vi "test.vi"() -> ()   [LabVIEW 2023, in "Serial_communication.lvlib"]
uses:
  Serial_communication.lvlib
panel:
  out "Read value 2":string
  out "LED ON":bool
  in  "?":bool
  out "Read value":string
  in  "stop":bool
  in  "Command":string
  in  "?":bool
  out "error out":errorcluster
  in  "Visa resourse":refnum<visa-resource-name>
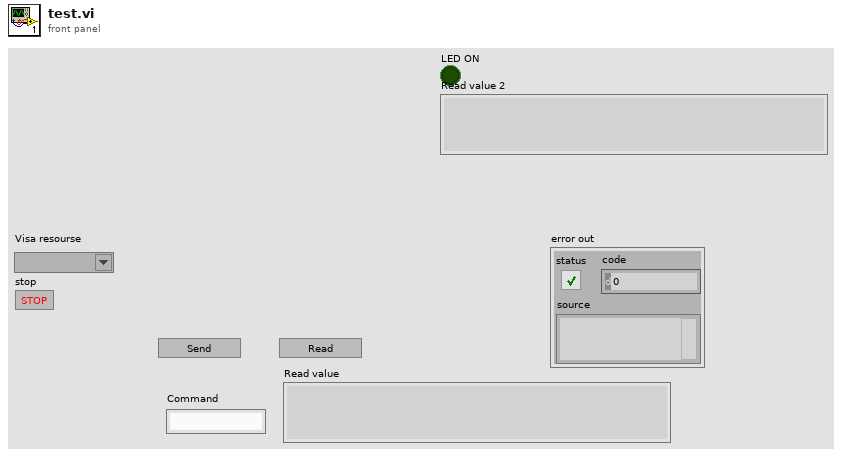
[diagram p1: front panel]
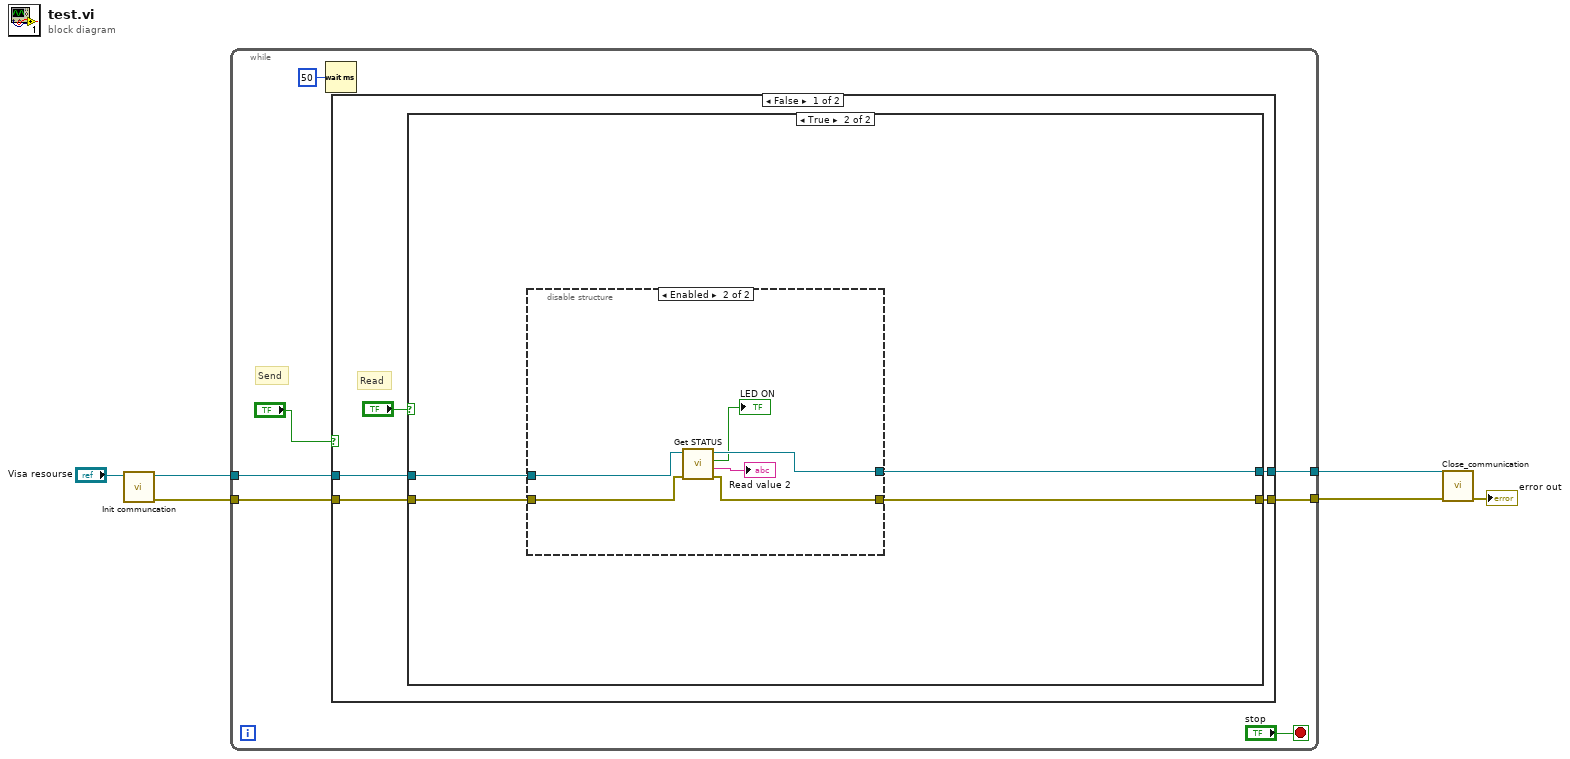
[diagram p0: block diagram]
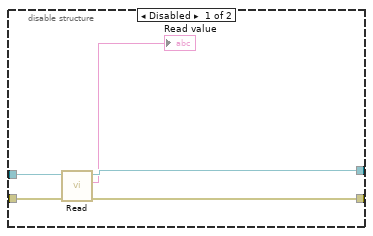
[diagram p3: hidden frame]
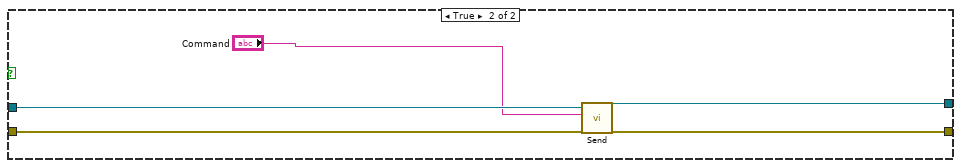
[diagram p4: hidden frame]
diagram:
  n1 = call "Init communcation.vi"("COM port"="Visa resourse") -> ("error out"=w3:errorcluster, "VISA Refnum out"=w4:refnum<visa-resource-name>)  [unwired: 9 in]
  n2 = while {
    tunnel: w4 -> [w12]
    tunnel: w3 -> [w11]
    tunnel: [w8] -> w2
    tunnel: [w7] -> w1
    stop <- "stop" stop-if-true
    # "Send"
    n3 = Wait (ms)(milliseconds to wait=u32 50) -> ()  [unwired: 1 out]
    n4 = case shown="False" "?" {
      tunnel: w12 -> [w18 w40]
      tunnel: w11 -> [w17 w39]
      tunnel: [w16 w38] -> w8
      tunnel: [w15 w37] -> w7
      frame False {
        # "Read"
        n5 = case shown="True" "?" {
          tunnel: w18 -> [w19 w24]
          tunnel: w17 -> [w20 w23]
          tunnel: [w19 w22] -> w16
          tunnel: [w20 w21] -> w15
          frame False {
          }
          frame True {
            n6 = disable-structure shown="Enabled" {
              disable-tunnel: w24 -> [w29 w35]
              disable-tunnel: w23 -> [w28 w34]
              disable-tunnel: [w27 w33] -> w22
              disable-tunnel: [w26 w32] -> w21
              frame Disabled {
                n7 = call "Read.vi"("error in (no error)"=w28, "VISA Refnum in"=w29) -> ("error out"=w26:errorcluster, "Read value"=→"Read value":string, "VISA Refnum out"=w27:refnum<visa-resource-name>)  [unwired: 7 in]
              }
              frame Enabled {
                n8 = call "Get STATUS.vi"("error in (no error)"=w34, "VISA Refnum in"=w35) -> ("error out"=w32:errorcluster, "Read value"=→"Read value 2":string, "LED ON"=→"LED ON":bool, "VISA Refnum out"=w33:refnum<visa-resource-name>)  [unwired: 6 in]
              }
            }
          }
        }
      }
      frame True {
        n9 = call "Send.vi"("error in (no error)"=w39, "Command"="Command", "VISA Refnum in"=w40) -> ("error out"=w37:errorcluster, "VISA Refnum out"=w38:refnum<visa-resource-name>)  [unwired: 7 in]
      }
    }
  }
  n10 = call "Close_communication.vi"("error in (no error)"=w1, "VISA Refnum in"=w2) -> ("error out"=→"error out":errorcluster)  [unwired: 9 in]
